vi "2 Element Array Overflow Support FXP(+-,14,1).vi"(0 "data in":fxp<+/-,14,1>[](array[numeric])=[0.0, 0.0], 5 "overflow":bool) -> (4 "data out":fxp<+/-,14,1>[](array[numeric]))   [LabVIEW 2014]
doc: "Adds overflow to input data.\n\n<B>Supported data types</B>\nFXP +-,18,1; FXP +-,14,1\n\n<B>Supported channel size</B>\n4, 8\n\n<B>Supported samples per cycle</B>\n2\n\n<B>Input Parameters</B>\n\n<B>data in</B> specifies the data input without the overflow.\n\n<B>overflow</B> specifies the overflow to add to the input data.\n\n<B>Output Parameters</B>\n\n<B>data out</B> returns the data with overflow added."
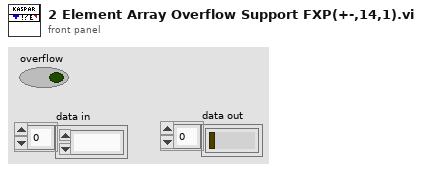
[diagram p1: front panel]
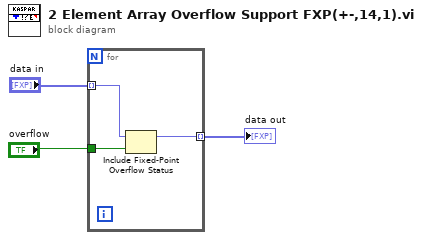
[diagram p0: block diagram]
diagram:
  n1 = for {
    tunnel: "overflow" -> [w6]
    tunnel: "data in" -> [w5] mode=indexing
    tunnel: [w4] -> w1 mode=indexing
    n2 = Include Fixed-Point Overflow Status(2:w6, 3:w5) -> (1:w4:fxp<+/-,14,1>)
  }
  "data out" <- w1
